vi "Simple_Calculator.vi"() -> ()   [LabVIEW 2022 SP3]
panel:
  out "?":bool
  out "Result":dbl
  in  "Operation":T1(ring)
  in  "Y":dbl
  in  "X":dbl
  # "Simple Calculator:\nEnter a value for both X and Y, then select an operation.\nThe result, assuming there is one will populate on the right."
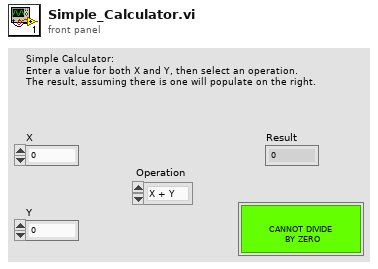
[diagram p1: front panel]
types:
  T1 = enum16{"X + Y", "X - Y", "X * Y", "X / Y", "X**Y"}
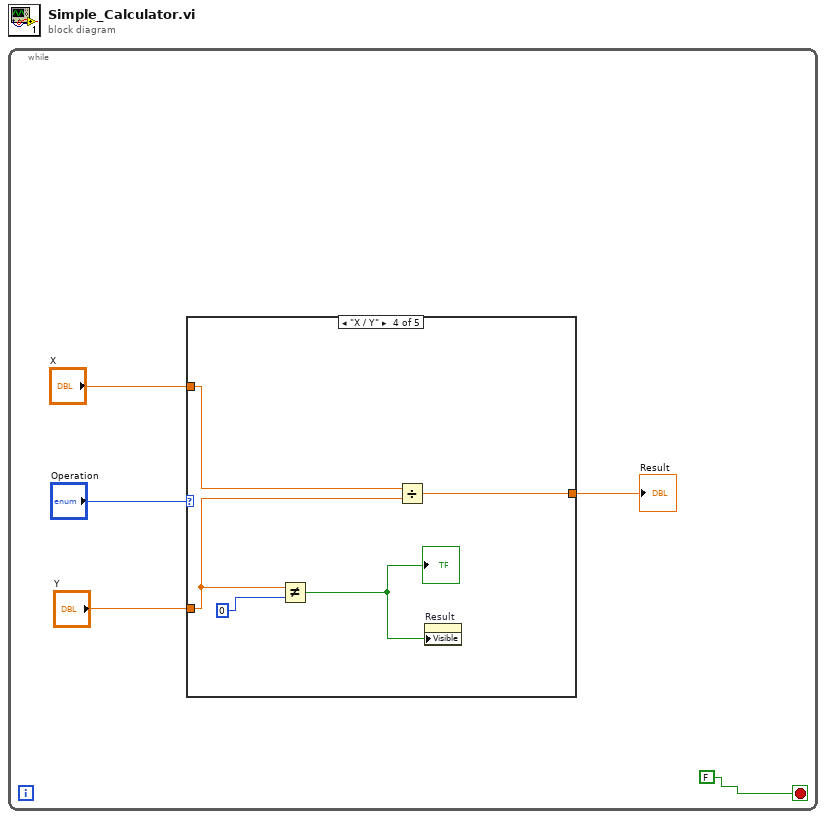
[diagram p0: block diagram]
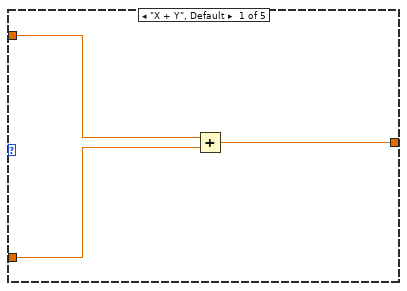
[diagram p2: hidden frame]
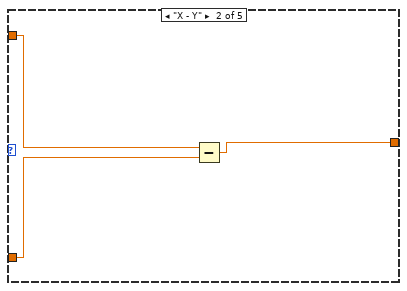
[diagram p3: hidden frame]
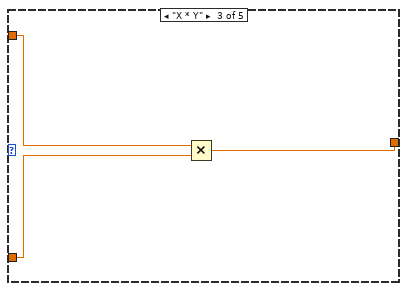
[diagram p4: hidden frame]
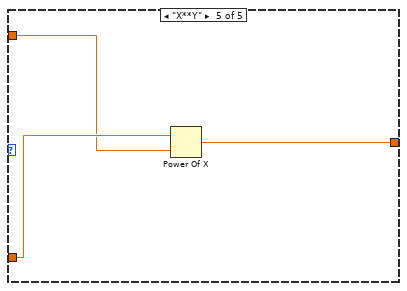
[diagram p5: hidden frame]
diagram:
  n1 = while {
    stop <- FALSE stop-if-true
    n2 = case shown="\"X / Y\"" "Operation" {
      tunnel: "X" -> [w8 w11 w14 w19 w21]
      tunnel: "Y" -> [w7 w10 w13 w17 w22]
      tunnel: [w6 w9 w12 w18 w20] -> w2
      frame "X + Y", Default {
        n3 = Add(x=w8, y=w7) -> (x+y=w6:dbl)
      }
      frame "X - Y" {
        n4 = Subtract(x=w11, y=w10) -> (x-y=w9:dbl)
      }
      frame "X * Y" {
        n5 = Multiply(x=w14, y=w13) -> (x*y=w12:dbl)
      }
      frame "X / Y" {
        n6 = Not Equal?(x=w17, y=0) -> (x != y?=w15:bool)
        "?" <- w15
        n7 = Divide(x=w19, y=w17) -> (x/y=w18:dbl)
        n8 = property on="Result" class="DigNum (strict)"("Visible"=w15) -> ()  [unwired: 2 in, 2 out]
      }
      frame "X**Y" {
        n9 = Power Of X(1:w21, 2:w22) -> (0:w20:dbl)
      }
    }
    "Result" <- w2
  }
